vi "h5_init.vi"(5 "options":string, 7 "var":string, 8 "error in (no error)":errorcluster, 10 "RID":string, 11 "files":path[](array[path])) -> (0 "error out":errorcluster)   [LabVIEW 2013, in "tools.lvlib"]
uses:
  <vilib>/UPVI/lvhdf5/file.llb/LVH5F Operation.ctl
  <vilib>/UPVI/lvhdf5/attribute.llb/Simple H5Awrite (Variant).vi
  <vilib>/UPVI/lvhdf5/attribute.llb/LVH5A Operation.ctl
  <vilib>/UPVI/lvhdf5/attribute.llb/Simple H5Awrite.xnode
  <vilib>/UPVI/lvhdf5/library.llb/HDF5 Ref.ctl
  tools.lvlib
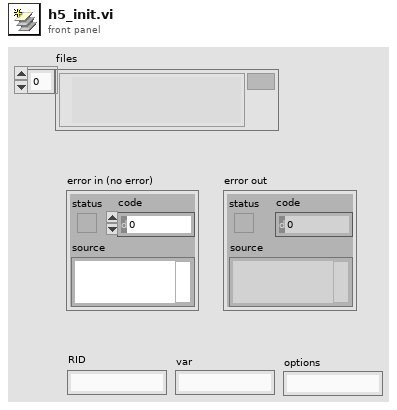
[diagram p1: front panel]
types:
  T1 = typedef "Semaphore RefNum" = refnum<k1>
  T2 = typedef "LVH5F Operation.ctl" = enum16{"open", "open or create", "create or replace", "create or replace (with confirmation)", "create", "open (read only)"}
  T3 = typedef "HDF5 Ref.ctl" = refnum<k1>
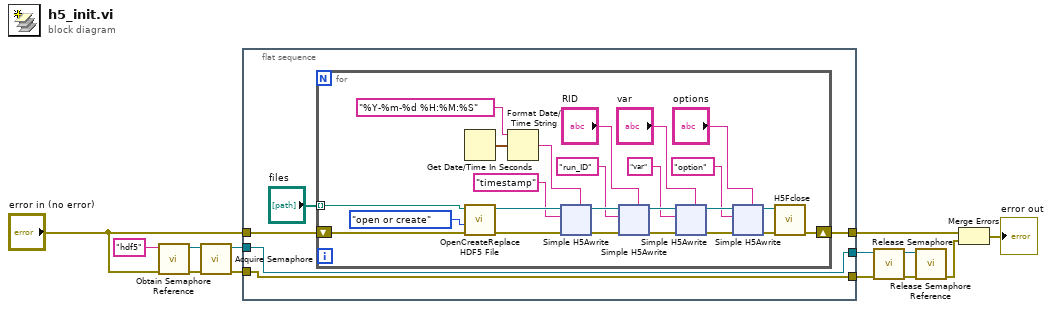
[diagram p0: block diagram]
diagram:
  n1 = call <vilib>:"Obtain Semaphore Reference.vi"("error in (no error)"="error in (no error)", "name (unnamed)"="hdf5") -> ("error out"=w12:errorcluster, "semaphore"=w13:T1)  [unwired: 3 in, 1 out]
  n2 = call <vilib>:"Acquire Semaphore.vi"("error in (no error)"=w12, "semaphore"=w13) -> ("error out"=w7:errorcluster, "semaphore out"=w6:T1)  [unwired: 3 in, 1 out]
  n3 = flat-sequence {
    tunnel: "error in (no error)" -> [w15]
    tunnel: w7 -> [w18]
    tunnel: w6 -> [w17]
    tunnel: [w18] -> w5
    tunnel: [w17] -> w4
    tunnel: [w16] -> w3
    frame #0 {
      n4 = for {
        shift-right: [w21] -> w16
        shift-left: w15 -> [w20]
        tunnel: "files" -> [w19] mode=indexing
        n5 = Get Date/Time In Seconds() -> (seconds since 1Jan1904=w38:timestamp)
        n6 = call <vilib>:"OpenCreateReplace HDF5 File.vi"("error in (no error)"=w20, "function (open or create)"=LVH5F_Operation."open or create", "path"=w19) -> ("error out"=w41:errorcluster, "HDF5 Ref out"=w42:T3)  [unwired: 5 in]
        n7 = Format Date/Time String(time format string (%c)="%Y-%m-%d %H:%M:%S", seconds (now)=w38) -> (date/time string=w37:string)  [unwired: 1 in]
        n8 = xnode "Simple H5Awrite"("HDF5 Ref"=w42, "Name"="timestamp", "error in (no error)"=w41, "Value"=w37) -> ("HDF5 Ref out"=w35:T3, "error out"=w29:errorcluster)  [unwired: 1 in]
        n9 = xnode "Simple H5Awrite"("HDF5 Ref"=w35, "Name"="run_ID", "error in (no error)"=w29, "Value"="RID") -> ("HDF5 Ref out"=w34:T3, "error out"=w30:errorcluster)  [unwired: 1 in]
        n10 = xnode "Simple H5Awrite"("HDF5 Ref"=w34, "Name"="var", "error in (no error)"=w30, "Value"="var") -> ("HDF5 Ref out"=w33:T3, "error out"=w31:errorcluster)  [unwired: 1 in]
        n11 = xnode "Simple H5Awrite"("HDF5 Ref"=w33, "Name"="option", "error in (no error)"=w31, "Value"="options") -> ("HDF5 Ref out"=w32:T3, "error out"=w28:errorcluster)  [unwired: 1 in]
        n12 = call <vilib>:"H5Fclose.vi"("error in (no error)"=w28, "HDF5 Ref"=w32) -> ("error out"=w21:errorcluster)  [unwired: 7 in]
      }
    }
  }
  n13 = call <vilib>:"Release Semaphore.vi"("error in (no error)"=w5, "semaphore"=w4) -> ("error out"=w10:errorcluster, "semaphore out"=w9:T1)  [unwired: 4 in]
  n14 = call <vilib>:"Release Semaphore Reference.vi"("error in (no error)"=w10, "semaphore"=w9) -> ("error out"=w2:errorcluster)  [unwired: 8 in, 1 out]
  n15 = Merge Errors(w3, w2) -> (→"error out":errorcluster)
